vi "Example Modbus Master.vi"() -> ()   [LabVIEW 2013]
uses:
  C:/tf/play/labview/Tinkerforge.dll
  Tinkerforge.dll
panel:
  out "message":string
  out "exceptionCode":i16
  out "requestID":u8
  in  "stop":bool
  in  "uid":string="amb"
  in  "port":i32=4223
  in  "host":string="localhost"
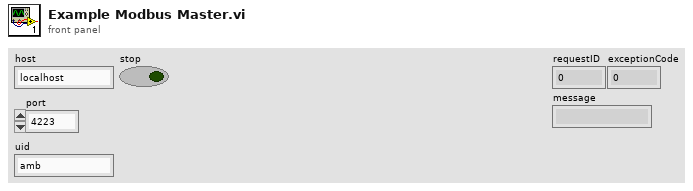
[diagram p1: front panel]
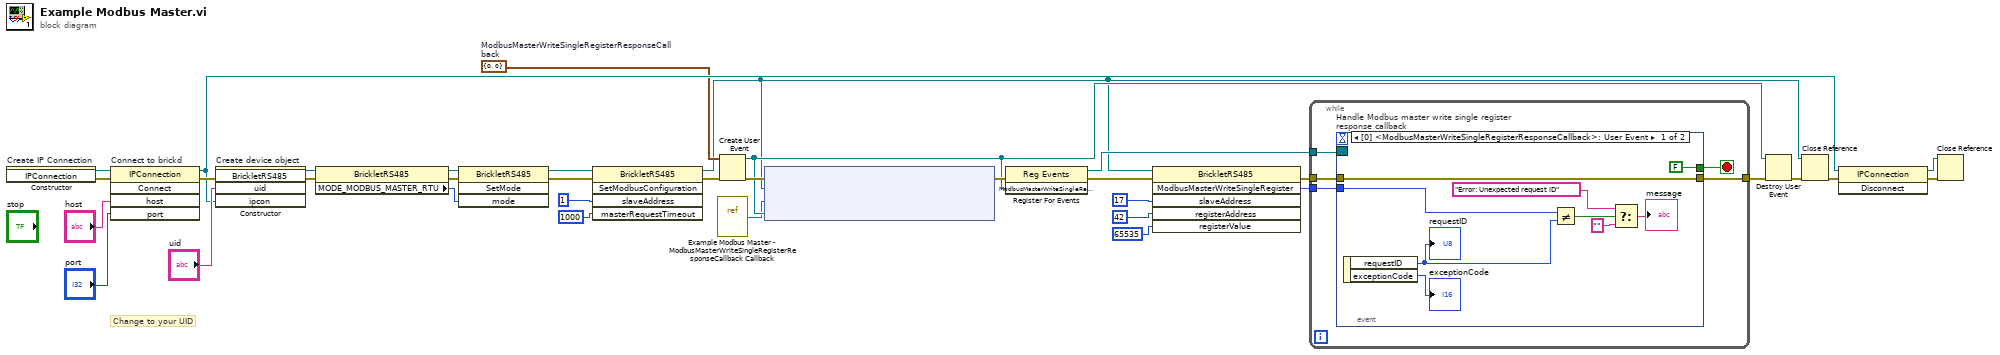
[diagram p0: block diagram]
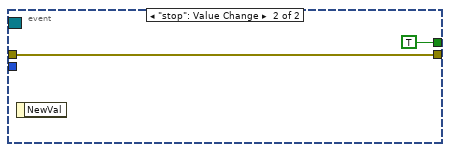
[diagram p2: hidden frame]
diagram:
  w19 = cluster{"requestID":u8, "exceptionCode":i16} {"requestID"=0, "exceptionCode"=0}  # ModbusMasterWriteSingleRegisterResponseCallback
  # "Change to your UID"
  n1 = constructor on="Create IP Connection" class="IPConnection"() -> (reference out=w35:refnum<k24>, error out=w20:errorcluster)  [unwired: 3 in, 1 out]
  n2 = invoke on="Connect to brickd" class="IPConnection" method="Connect"(reference=w35, error in=w20, "host"="host", "port"="port") -> (reference out=w28:refnum<k24>, error out=w31:errorcluster)  [unwired: 1 in, 3 out]
  n3 = constructor on="Create device object" class="BrickletRS485"(error in=w31, "uid"="uid", "ipcon"=w28) -> (reference out=w17:refnum<k24>, error out=w16:errorcluster)  [unwired: 2 in, 3 out]
  n4 = property class="BrickletRS485"(reference=w17, error in=w16) -> (reference out=w14:refnum<k24>, error out=w15:errorcluster, "MODE_MODBUS_MASTER_RTU"=w13:u8)
  n5 = invoke class="BrickletRS485" method="SetMode"(reference=w14, error in=w15, "mode"=w13) -> (reference out=w12:refnum<k24>, error out=w10:errorcluster)  [unwired: 1 in, 2 out]
  n6 = invoke class="BrickletRS485" method="SetModbusConfiguration"(reference=w12, error in=w10, "slaveAddress"=u8 1, "masterRequestTimeout"=i64 1000) -> (reference out=w6:refnum<k24>, error out=w11:errorcluster)  [unwired: 1 in, 3 out]
  n7 = vi-ref "Example Modbus Master - ModbusMasterWriteSingleRegisterResponseCallback Callback.vi"() -> ("vi reference"=w2:refnum<vi>)
  n8 = Create User Event(user event datatype=w19, error in=w11) -> (user event=w22:refnum<user-event>, error out=w26:errorcluster)
  n9 = node ("Register Event Callback")(w26, w6, w2, w22) -> (w25:errorcluster)  [unwired: 1 in, 1 out]
  n10 = register-events(error in=w25, w22) -> (reference out=w24:refnum<event-registration>, error out=w7:errorcluster)  [unwired: 1 in]
  n11 = invoke class="BrickletRS485" method="ModbusMasterWriteSingleRegister"(reference=w6, error in=w7, "slaveAddress"=u8 17, "registerAddress"=i64 42, "registerValue"=65535) -> (error out=w18:errorcluster, "ModbusMasterWriteSingleRegister"=w1:u8)  [unwired: 1 in, 4 out]
  n12 = while {
    tunnel: w24 -> [w37]
    tunnel: [w40] -> w23
    tunnel: w18 -> [w39]
    tunnel: w1 -> [w36]
    stop <- w38 stop-if-true
    n13 = event "Handle Modbus master write single register response callback" shown="[0] <ModbusMasterWriteSingleRegisterResponseCallback>: User Event" {
      selector: w37 -> [_ _]
      dyn-events: _ -> [_ _]
      timeout: _ -> [_ _]
      tunnel: [w49 w50] -> w40
      tunnel: w39 -> [w49 w50]
      tunnel: [FALSE TRUE] -> w38
      tunnel: w36 -> [w46 _]
      event User Event {
        n14 = event-data() -> ("requestID"=w47:u8, "exceptionCode"=→"exceptionCode":i16)  [unwired: 1 in]
        "requestID" <- w47
        n15 = Not Equal?(x=w46, y=w47) -> (x != y?=w44:bool)
        n16 = Select(t="Error: Unexpected request ID", s=w44, f="") -> (s? t:f=→"message":string)
      }
      event "stop": Value Change {
        n17 = event-data() -> ()  [unwired: 1 in, 1 out]
      }
    }
  }
  n18 = Destroy User Event(user event=w22, error in=w23) -> (error out=w21:errorcluster)
  n19 = Close Reference(reference=w6, error in (no error)=w21) -> (error out=w30:errorcluster)
  n20 = invoke class="IPConnection" method="Disconnect"(reference=w28, error in=w30) -> (reference out=w27:refnum<k24>, error out=w29:errorcluster)  [unwired: 1 in, 1 out]
  n21 = Close Reference(reference=w27, error in (no error)=w29) -> ()  [unwired: 1 out]
